vi "Port Init.vi"(8 "error in (no error)":errorcluster caption="error in（no error）", 11 "Port Selection Info In":T1={"Port Name"="", "Amplifier Num"=1, "Baud Rate"=38400, "Char Formation"=enum."0"} {"Baud Rate" items=["38400"=38400, "19200"=19200, "9600"=9600, "115200"=0]; "Amplifier Num" max=31}) -> (0 "error out":errorcluster, 3 "Port Selection Info Out":T1={"Port Name"="", "Amplifier Num"=1, "Baud Rate"=38400, "Char Formation"=enum."0"} {"Baud Rate" items=["38400"=38400, "19200"=19200, "9600"=9600, "115200"=0]; "Amplifier Num" max=31})   [LabVIEW 2014, in "ALPHA5 RS485.lvlib"]
uses:
  ALPHA5 RS485.lvlib
  typedefs/Port Selection Info.ctl
  <vilib>/Instr/_visa.llb/VISA Flush IO Buffer Mask.ctl
  <vilib>/Instr/_visa.llb/VISA Configure Serial Port (Instr).vi
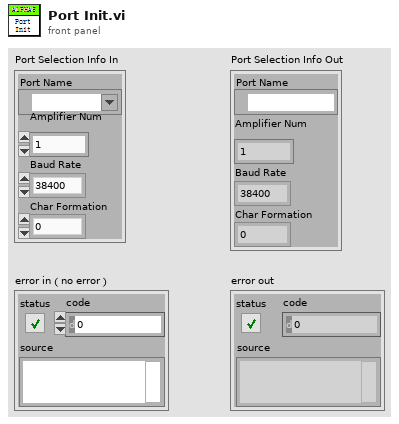
[diagram p1: front panel]
types:
  T1 = typedef "ALPHA5 RS485.lvlib/Port Selection Info.ctl" = cluster{"Port Name":refnum<visa-resource-name>, "Amplifier Num":u8, "Baud Rate":u32, "Char Formation":enum16{"0", "1", "2", "3", "4", "5"}}
  T2 = typedef "VISA Flush IO Buffer Mask.ctl" = u16
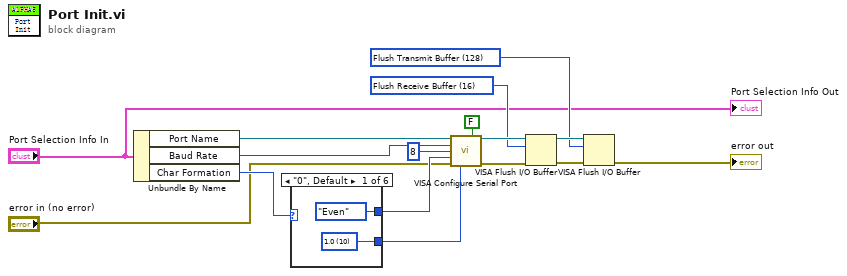
[diagram p0: block diagram]
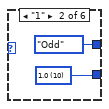
[diagram p2: hidden frame]
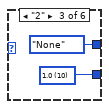
[diagram p3: hidden frame]
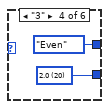
[diagram p4: hidden frame]
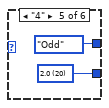
[diagram p5: hidden frame]
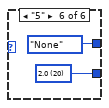
[diagram p6: hidden frame]
diagram:
  w6 = T2 128 items=["Flush Receive Buffer"=16, "Write Transmit Buffer to Device"=32, "Flush Receive Buffer (No I/O)"=64, "Flush Transmit Buffer"=128] ("Mask")
  w8 = T2 16 items=["Flush Receive Buffer"=16, "Write Transmit Buffer to Device"=32, "Flush Receive Buffer (No I/O)"=64, "Flush Transmit Buffer"=128] ("Mask")
  n1 = Unbundle By Name("Port Selection Info In") -> ("Port Name"=w16:refnum<visa-resource-name>, "Baud Rate"=w15:u32, "Char Formation"=w14:enum16{"0", "1", "2", "3", "4", "5"})
  n2 = case shown="\"0\", Default" w14 {
    tunnel: [enum16{"None", "Odd", "Even", "Mark", "Space"}."Even" ("parity (0:none)") enum16{"None", "Odd", "Even", "Mark", "Space"}."Odd" ("parity (0:none)") enum16{"None", "Odd", "Even", "Mark", "Space"}."None" ("parity (0:none)") enum16{"None", "Odd", "Even", "Mark", "Space"}."Even" ("parity (0:none)") enum16{"None", "Odd", "Even", "Mark", "Space"}."Odd" ("parity (0:none)") enum16{"None", "Odd", "Even", "Mark", "Space"}."None" ("parity (0:none)")] -> w11
    tunnel: [w17 w19 w21 w23 w25 w27] -> w10
    frame "0", Default {
      w17 = u16 10 items=["1.0"=10, "1.5"=15, "2.0"=20] ("stop bits (10: 1 bit)")
    }
    frame "1" {
      w19 = u16 10 items=["1.0"=10, "1.5"=15, "2.0"=20] ("stop bits (10: 1 bit)")
    }
    frame "2" {
      w21 = u16 10 items=["1.0"=10, "1.5"=15, "2.0"=20] ("stop bits (10: 1 bit)")
    }
    frame "3" {
      w23 = u16 20 items=["1.0"=10, "1.5"=15, "2.0"=20] ("stop bits (10: 1 bit)")
    }
    frame "4" {
      w25 = u16 20 items=["1.0"=10, "1.5"=15, "2.0"=20] ("stop bits (10: 1 bit)")
    }
    frame "5" {
      w27 = u16 20 items=["1.0"=10, "1.5"=15, "2.0"=20] ("stop bits (10: 1 bit)")
    }
  }
  n3 = call-poly "VISA Configure Serial Port"("VISA resource name"=w16, "Enable Termination\nChar (T)"=FALSE ("Enable Termination\nChar (T)"), "baud rate (9600)"=w15, "data bits (8)"=u16 8, "parity (0:none)"=w11, "error in (no error)"="error in (no error)", "stop bits (10: 1 bit)"=w10) -> ("VISA resource name out"=w9:refnum<visa-resource-name>, "error out"=w5:errorcluster)  [unwired: 7 in]
  n4 = VISA Flush I/O Buffer(VISA resource name=w9, mask (16)=w8, error in (no error)=w5) -> (VISA resource name out=w7:refnum<visa-resource-name>, error out=w4:errorcluster)
  n5 = VISA Flush I/O Buffer(VISA resource name=w7, mask (16)=w6, error in (no error)=w4) -> (error out=→"error out":errorcluster)  [unwired: 1 out]
  "Port Selection Info Out" <- "Port Selection Info In"
